vi "pathfinder prepare.vi"(0 "path":T1[](array[typedef]), 1 "sample_count":i32=10000, 5 "max_velocity":dbl, 7 "max_acceleration":dbl, 9 "max_jerk":dbl, 11 "error in (no error)":errorcluster, 12 "dt":dbl) -> (4 "function return":i32, 15 "error out":errorcluster)   [LabVIEW 2016, in "Pathfinder.lvlib"]
doc: "CAPI int pathfinder_prepare_LabVIEW(const Waypoint *path, int path_length, int sample_count, double dt,\n double max_velocity, double max_acceleration, double max_jerk);"
uses:
  Pathfinder.lvlib
  Waypoint.ctl
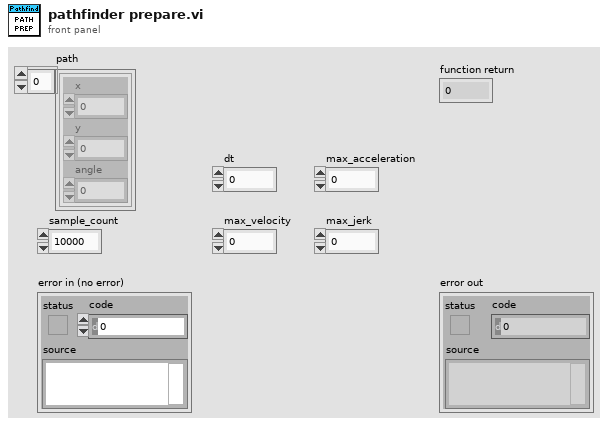
[diagram p1: front panel]
types:
  T1 = typedef "Pathfinder.lvlib/Waypoint.ctl" = cluster{"x":dbl, "y":dbl, "angle":dbl}
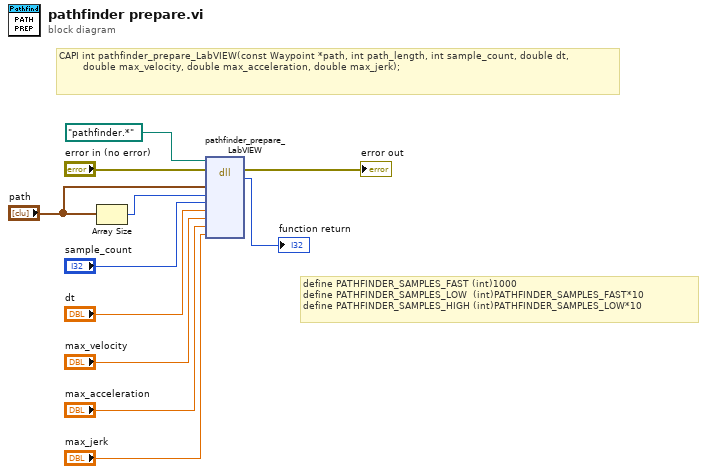
[diagram p0: block diagram]
diagram:
  # "define PATHFINDER_SAMPLES_FAST (int)1000\ndefine PATHFINDER_SAMPLES_LOW  (int)PATHFINDER_SAMPLES_FAST*10\ndefine PATHFINDER_SAMPLES_HIGH (int)PATHFINDER_SAMPLES_LOW*10"
  # "CAPI int pathfinder_prepare_LabVIEW(const Waypoint *path, int path_length, int sample_count, double dt,\n        double max_velocity, double max_acceleration, double max_jerk);"
  n1 = Array Size(array="path") -> (size(s)=w4:i32)
  n2 = dll-call lib="?" fn="pathfinder_prepare_LabVIEW"(path in=path "pathfinder.*", error in="error in (no error)", "path"="path", "path_length"=w4, "sample_count"="sample_count", "dt"="dt", "max_velocity"="max_velocity", "max_acceleration"="max_acceleration", "max_jerk"="max_jerk") -> (error out=→"error out":errorcluster, "return type"=→"function return":i32)  [unwired: 8 in, 1 out]
